vi "Inverse Kinematics.vi"(6 "r(m)":dbl, 8 "L(m)":dbl, 9 "Theta Set":dbl, 10 "Y Set":dbl, 11 "X Set":dbl) -> (1 "Out Motor 3":dbl, 2 "Out Motor 2":dbl, 3 "Out Motor 1":dbl)   [LabVIEW 2019]
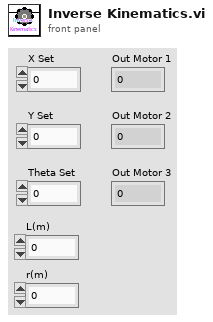
[diagram p1: front panel]
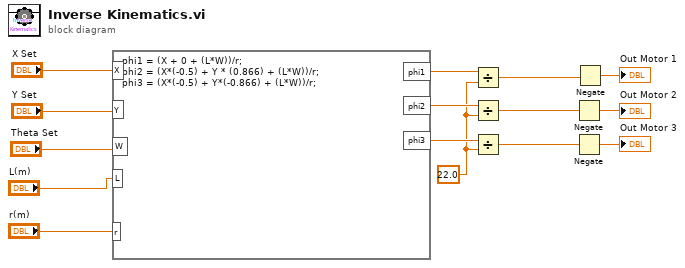
[diagram p0: block diagram]
diagram:
  w7 = 22.0 ("y")
  # "L =  0.8354\nr = 0.0355"
  n1 = formula code="phi1 = (X + 0 + (L*W))/r;\nphi2 = (X*(-0.5) + Y * (0.866) + (L*W))/r;\nphi3 = (X*(-0.5) + Y*(-0.866) + (L*W))/r;"("X"="X Set", "Y"="Y Set", "W"="Theta Set", "L"="L(m)", "r"="r(m)") -> ("phi1"=w10:dbl, "phi2"=w9:dbl, "phi3"=w8:dbl)
  n2 = Divide(x=w10, y=w7) -> (x/y=w4:dbl)
  n3 = Divide(x=w9, y=w7) -> (x/y=w3:dbl)
  n4 = Divide(x=w8, y=w7) -> (x/y=w2:dbl)
  n5 = Negate(x=w3) -> (-x=→"Out Motor 2":dbl)
  n6 = Negate(x=w2) -> (-x=→"Out Motor 3":dbl)
  n7 = Negate(x=w4) -> (-x=→"Out Motor 1":dbl)
